vi "Write Control Refnum.vi"(10 "Ctl Refnum":refnum<vi>, 11 "TerminalReference in":refnum<class "TerminalPropertyBinding.lvclass">) -> (3 "TerminalReferenceBinding Out":refnum<class "TerminalPropertyBinding.lvclass">)   [LabVIEW 2018, in "MVA Framework.lvlib" / "TerminalPropertyBinding.lvclass"]
doc: "写入控件引用"
uses:
  TerminalPropertyBinding.lvclass
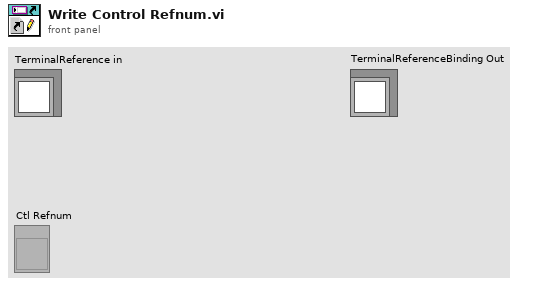
[diagram p1: front panel]
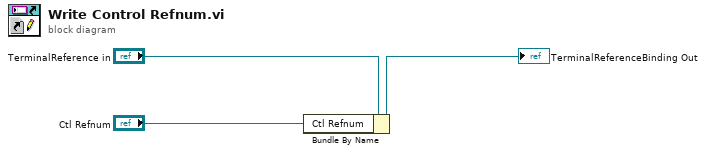
[diagram p0: block diagram]
diagram:
  n1 = Bundle By Name(cluster="TerminalReference in", "Ctl Refnum"="Ctl Refnum") -> (→"TerminalReferenceBinding Out":refnum<class "TerminalPropertyBinding.lvclass">)
